vi "Sync Minor Frame Messages.vi"(8 "error in (no error)":errorcluster, 11 "Major Frame in":refnum<class "Major Frame.lvclass">) -> (0 "error out":errorcluster, 3 "Major Frame out":refnum<class "Major Frame.lvclass">)   [LabVIEW 2020, in "BCI-1553 API.lvlib" / "Major Frame.lvclass"]
doc: "Forces all the minor frames to have a copy of the message list owned by the major frame. Another step to make sure that only one instance of a message is ever instantiated."
uses:
  Major Frame.lvclass
  Major Frame.lvclass/Major Frame.ctl
  Minor Frame/Minor Frame.lvclass
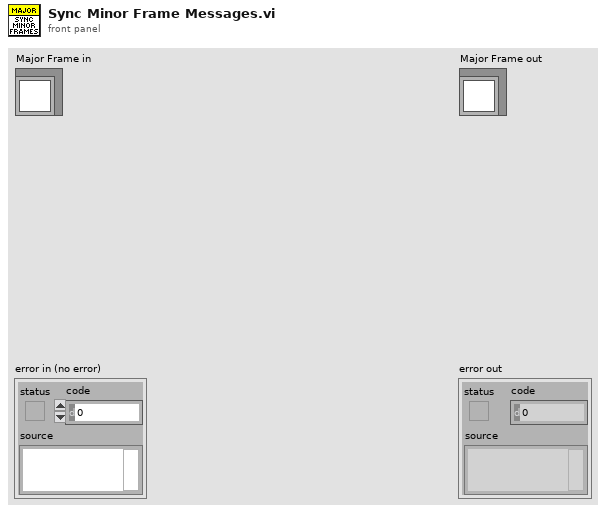
[diagram p1: front panel]
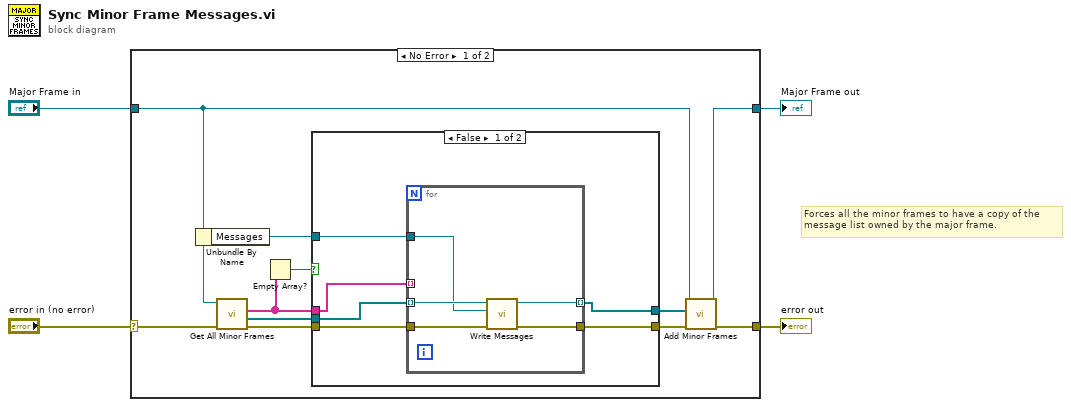
[diagram p0: block diagram]
diagram:
  # "Forces all the minor frames to have a copy of the\nmessage list owned by the major frame."
  n1 = case shown="No Error" "error in (no error)" {
    selector: "error in (no error)" -> [w15 w30]
    tunnel: [w6 w30] -> w3
    tunnel: [w8 w29] -> w1
    tunnel: "Major Frame in" -> [w9 w29]
    frame No Error {
      n2 = Unbundle By Name(w9) -> ("Messages"=w11:refnum<class "Registry.lvclass">)
      n3 = call-dynamic "Get All Minor Frames.vi"("error in (no error)"=w15, "Major Frame in"=w9) -> ("error out"=w10:errorcluster, "Minor Frames"=w13:refnum<class "Minor Frame.lvclass">[], "Minor Frame IDs"=w12:string[])  [unwired: 6 in, 1 out]
      n4 = Empty Array?(array=w12) -> (empty?=w14:bool)
      n5 = case shown="False" w14 {
        tunnel: w13 -> [w19 w27]
        tunnel: w12 -> [w17 _]
        tunnel: w11 -> [w18 _]
        tunnel: w10 -> [w21 w28]
        tunnel: [w20 w28] -> w5
        tunnel: [w16 w27] -> w7
        frame False {
          n6 = for {
            tunnel: w21 -> [w26]
            tunnel: [w25] -> w20
            tunnel: w19 -> [w24] mode=indexing
            tunnel: w18 -> [w22]
            tunnel: [w23] -> w16 mode=indexing
            tunnel: w17 -> [_] mode=indexing
            n7 = call-dynamic "Write Messages.vi"("error in (no error)"=w26, "Messages"=w22, "Minor Frame in"=w24) -> ("error out"=w25:errorcluster, "Minor Frame out"=w23:refnum<class "Minor Frame.lvclass">)  [unwired: 7 in]
          }
        }
        frame True {
        }
      }
      n8 = call-dynamic "Add Minor Frames.vi"("error in (no error)"=w5, "Minor Frames"=w7, "Major Frame in"=w9) -> ("error out"=w6:errorcluster, "Major Frame out"=w8:refnum<class "Major Frame.lvclass">)  [unwired: 7 in]
    }
    frame Error {
    }
  }
  "error out" <- w3
  "Major Frame out" <- w1
